vi "菜单-另存为.vi"(8 "error in (no error)":errorcluster caption="错误输入（无错误）", 11 "程序响应 输入":refnum<class "程序响应.lvclass">) -> (0 "error out":errorcluster caption="错误输出", 3 "程序响应 输出":refnum<class "程序响应.lvclass">)   [LabVIEW 2020, in "程序响应.lvlib" / "程序响应.lvclass"]
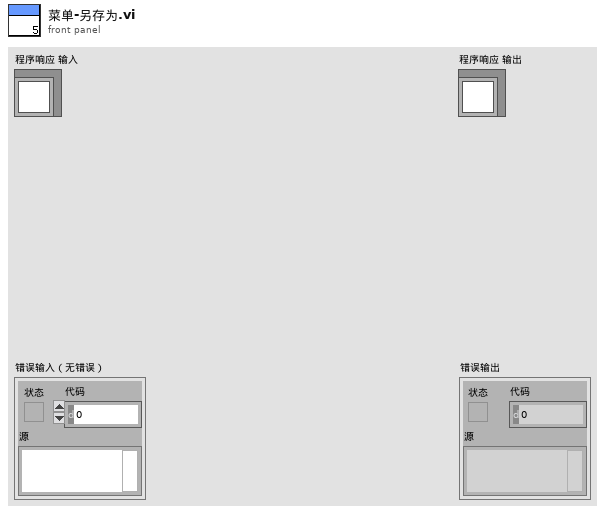
[diagram p1: front panel]
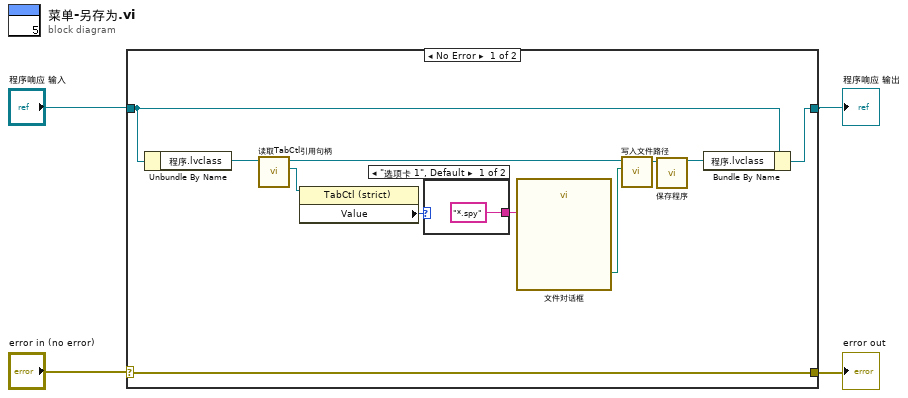
[diagram p0: block diagram]
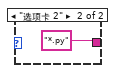
[diagram p2: hidden frame]
diagram:
  n1 = case shown="No Error" "error in (no error)" {
    selector: "error in (no error)" -> [w15 w19]
    tunnel: [w15 w19] -> w1
    tunnel: [w12 w18] -> w4
    tunnel: "程序响应 输入" -> [w13 w18]
    frame No Error {
      n2 = Unbundle By Name(w13) -> ("程序.lvclass"=w6:refnum<class "程序.lvclass">)
      n3 = call-dynamic "读取TabCtl引用句柄.vi"("程序输入"=w6) -> ("TabCtl引用句柄"=w8:refnum<vi>, "程序输出"=w5:refnum<class "程序.lvclass">)  [unwired: 8 in, 1 out]
      n4 = property class="TabCtl (strict)"(reference=w8) -> ("Value"=w9:enum32{"选项卡 1", "选项卡 2"})  [unwired: 1 in, 2 out]
      n5 = case shown="\"选项卡 1\", Default" w9 {
        tunnel: ["*.spy" ("pattern (all files)") "*.py" ("pattern (all files)")] -> w7
        frame "选项卡 1", Default {
        }
        frame "选项卡 2" {
        }
      }
      n6 = call "文件对话框"("pattern (all files)"=w7) -> ("selected path"=w10:path)  [unwired: 11 in, 3 out]
      n7 = call-dynamic "写入文件路径.vi"("文件路径"=w10, "程序输入"=w5) -> ("程序输出"=w11:refnum<class "程序.lvclass">)  [unwired: 8 in, 1 out]
      n8 = call-dynamic "保存程序.vi"("程序 输入"=w11) -> ("程序 输出"=w14:refnum<class "程序.lvclass">)  [unwired: 9 in, 1 out]
      n9 = Bundle By Name(cluster=w13, "程序.lvclass"=w14) -> (w12:refnum<class "程序响应.lvclass">)
    }
    frame Error {
    }
  }
  "error out" <- w1
  "程序响应 输出" <- w4
